vi "sr_war.vi"() -> ()   [LabVIEW 2025]
panel:
  out "wariancja":dbl
  out "œrednia":dbl
  in  "offset":dbl
  in  "Sygnal":T1(ring)
  in  "freq":dbl
  in  "phase":dbl
  in  "Amp":dbl
  in  "stop":bool
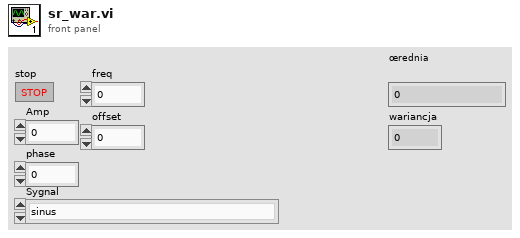
[diagram p1: front panel]
types:
  T1 = enum16{"sinus", "prostokat", "pila", "trojkat", "rozklad losowy", "rozklad normalny"}
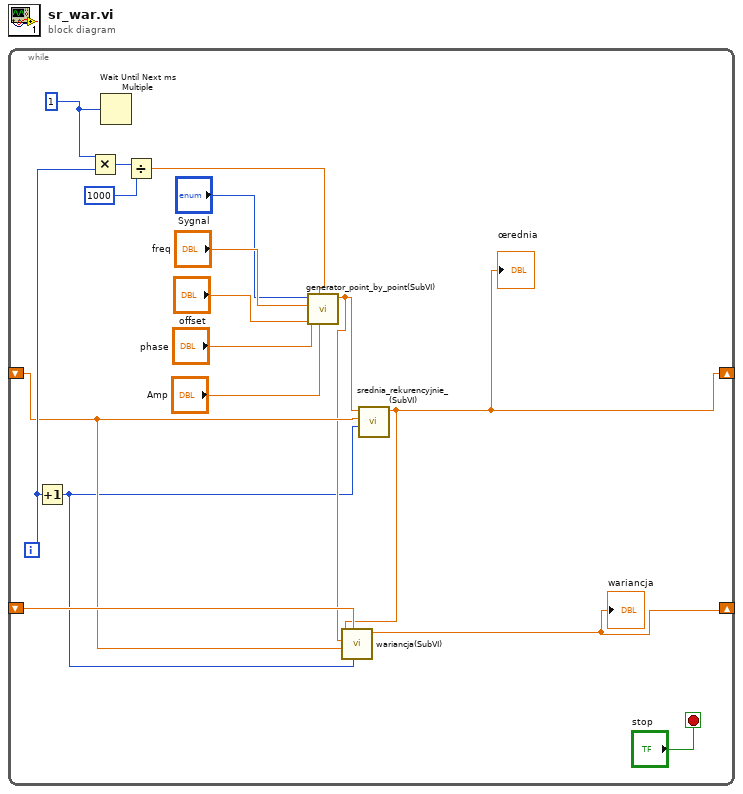
[diagram p0: block diagram]
diagram:
  n1 = while {
    shift-right: [w5] -> _
    shift-left: _ -> [w4]
    shift-right: [w1] -> _
    shift-left: _ -> [w6]
    i -> [w7]
    stop <- "stop" stop-if-true
    w11 = u32 1 ("millisecond multiple")
    n2 = Increment(x=w7) -> (x+1=w2:i32)
    n3 = Multiply(x=w11, y=w7) -> (x*y=w10:u32)
    n4 = Wait Until Next ms Multiple(millisecond multiple=w11) -> ()  [unwired: 1 out]
    n5 = Divide(x=w10, y=u32 1000) -> (x/y=w8:dbl)
    n6 = call "generator_point_by_point(SubVI).vi"("Amp"="Amp", "Numeric"=w8, "offset"="offset", "phase"="phase", "freq"="freq", "Sygnal"="Sygnal") -> ("Gaussian white noise"=w3:dbl)  [unwired: 5 in]
    n7 = call "srednia_rekurencyjnie_(SubVI).vi"("N"=w2, "œr N-1"=w4, "Gaussian white noise"=w3) -> ("œrednia"=w5:dbl)  [unwired: 8 in]
    "œrednia" <- w5
    n8 = call "wariancja(SubVI).vi"("iteracja N"=w2, "wariancja N-1"=w6, "œrednia N-1"=w4, "Gaussian white noise"=w3, "œrednia N"=w5) -> ("wariancja"=w1:dbl)  [unwired: 6 in]
    "wariancja" <- w1
  }
